vi "datacodecomb.vi"(5 "数据精度":i32=6, 6 "字段结束":bool=TRUE, 7 "数据标识":string="N", 8 "数据类型":string(combo)="-Rtd=", 9 "污染物编码":string, 10 "地表水/污染源":bool, 11 "污染物浓度":string) -> (0 "编码输出":string)   [LabVIEW 2016, in "212format_work.lvclass"]
uses:
  212format_work.lvclass
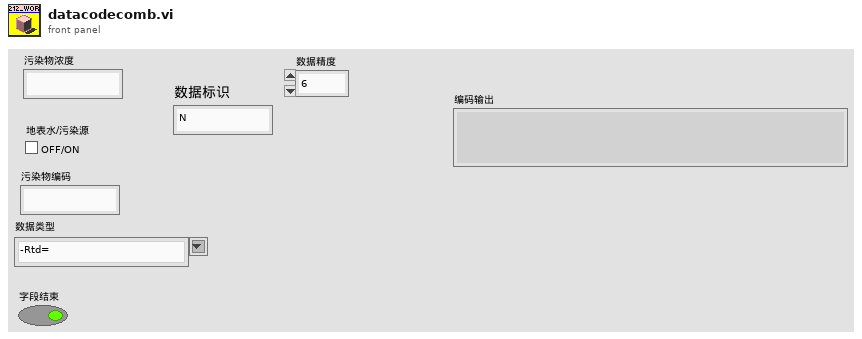
[diagram p1: front panel]
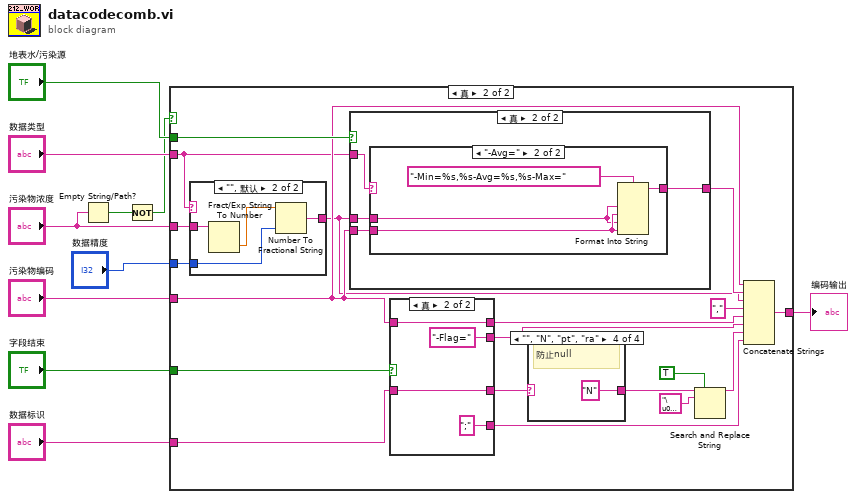
[diagram p0: block diagram]
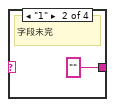
[diagram p7: hidden frame]
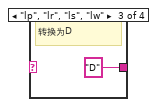
[diagram p8: hidden frame]
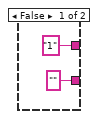
[diagram p9: hidden frame]
diagram:
  n1 = Empty String/Path?(string/path="污染物浓度") -> (empty?=w4:bool)
  n2 = Not(x=w4) -> (.not. x?=w2:bool)
  n3 = case shown="真" w2 {
    tunnel: [_ w28] -> w10
    tunnel: "字段结束" -> [_ w26]
    tunnel: "地表水/污染源" -> [_ w18]
    tunnel: "数据类型" -> [_ w14]
    tunnel: "污染物编码" -> [_ w17]
    tunnel: "数据标识" -> [_ w15]
    tunnel: "污染物浓度" -> [_ w13]
    tunnel: "数据精度" -> [_ w11]
    frame False {
    }
    frame True {
      n4 = case shown="\"\", 默认" w14 {
        tunnel: w13 -> [w30 w33]
        tunnel: [w30 w32] -> w12
        tunnel: w11 -> [_ w31]
        frame "-WaterTime=" {
        }
        frame "", Default {
          n5 = Fract/Exp String To Number(string=w33) -> (number=w34:dbl)  [unwired: 3 in, 1 out]
          n6 = Number To Fractional String(number=w34, precision (6)=w31) -> (F-format string=w32:string)  [unwired: 2 in]
        }
      }
      n7 = case shown="真" w18 {
        tunnel: w14 -> [w35 w39]
        tunnel: [w35 w38] -> w16
        tunnel: w17 -> [_ w37]
        tunnel: w12 -> [_ w36]
        frame False {
        }
        frame True {
          n8 = case shown="\"-Avg=\"" w39 {
            selector: w39 -> [w40 _]
            tunnel: [w40 w41] -> w38
            tunnel: w37 -> [_ w43]
            tunnel: w36 -> [_ w42]
            frame "假", Default {
            }
            frame "-Avg=" {
              n9 = Format Into String(format string="-Min=%s,%s-Avg=%s,%s-Max=" ("格式字符串"), w42, w43, w42, w43) -> (resulting string=w41:string)  [unwired: 2 in, 1 out]
            }
          }
        }
      }
      n10 = case shown="真" w26 {
        tunnel: [_ "-Flag=" ("字符串")] -> w27
        tunnel: ["1" ("字符串") w51] -> w24
        tunnel: w17 -> [_ w53]
        tunnel: [_ w53] -> w25
        tunnel: ["" ("字符串") ";" ("字符串")] -> w19
        tunnel: w15 -> [_ w51]
        frame False {
        }
        frame True {
        }
      }
      n11 = case shown="\"\", \"N\", \"pt\", \"ra\"" w24 {
        selector: w24 -> [w45 _ _ _]
        tunnel: [w45 "" ("字符串") "D" ("字符串") "N" ("字符串")] -> w23
        frame Default {
          # "其他透传"
        }
        frame "1" {
          # "字段未完"
        }
        frame "lp", "lr", "ls", "lw" {
          # "转换为D"
        }
        frame "", "N", "pt", "ra" {
          # "防止null"
        }
      }
      n12 = Search and Replace String(replace all?=TRUE ("替换全部？(F)"), input string=w23, search string="\u0000" ("搜索字符串")) -> (result string=w21:string)  [unwired: 5 in, 3 out]
      n13 = Concatenate Strings(w17, w16, w12, "," ("字符串"), w25, w27, w21, w19) -> (w28:string)
    }
  }
  "编码输出" <- w10
